vi "Determine Mouse Down Action.vi"(8 "error in (no error)":errorcluster, 11 "DataGrid in":refnum<class "DataGrid.lvclass">) -> (0 "error out":errorcluster, 2 "Action":T1, 3 "DataGrid out":refnum<class "DataGrid.lvclass">)   [LabVIEW 2017, in "DataGrid.lvclass"]
uses:
  DataGrid.lvclass
  C:/Program Files (x86)/National Instruments/LabVIEW 2017/vi.lib/QSI/QControls/QControl Classes/MulticolumnListbox/MulticolumnListbox.lvclass
  Mouse Down Action.ctl
  Read Current Edit Position.vi
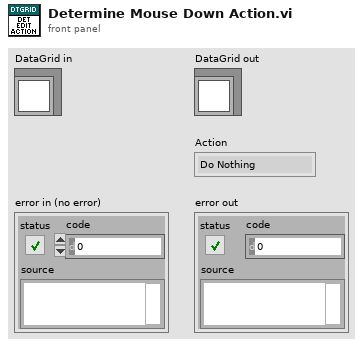
[diagram p1: front panel]
types:
  T1 = typedef "DataGrid.lvclass/Mouse Down Action.ctl" = enum16{"Do Nothing", "Sort Column", "Edit Only", "Add Row and Edit"}
  T2 = typedef "LVRowAndColumnTypeDef.ctl" = cluster{"Row":i32, "Column":i32}
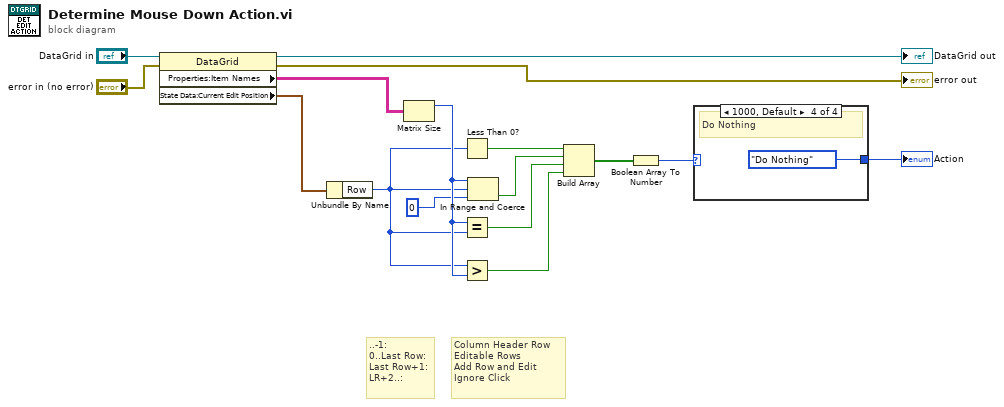
[diagram p0: block diagram]
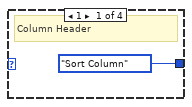
[diagram p2: hidden frame]
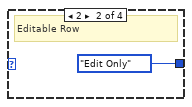
[diagram p3: hidden frame]
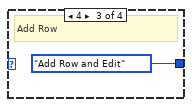
[diagram p4: hidden frame]
diagram:
  # "Column Header Row\nEditable Rows\nAdd Row and Edit\nIgnore Click"
  # "..-1:\n0..Last Row:\nLast Row+1:\nLR+2..:"
  n1 = property class="DataGrid"(reference="DataGrid in", error in="error in (no error)") -> (reference out=→"DataGrid out":refnum<class "DataGrid.lvclass">, error out=→"error out":errorcluster, "Properties:Item Names"=w13:string[][], "State Data:Current Edit Position"=w16:T2)
  n2 = Unbundle By Name(w16) -> ("Row"=w6:i32)
  n3 = Matrix Size(0:w13) -> (1:w7:i32)  [unwired: 1 out]
  n4 = Less Than 0?(x=w6) -> (x < 0?=w8:bool)
  n5 = Equal?(x=w7, y=w6) -> (x = y?=w10:bool)
  n6 = Greater?(x=w6, y=w7) -> (0:w11:bool)
  n7 = In Range and Coerce(upper limit=w7, x=w6, lower limit=0) -> (In Range?=w9:bool)  [unwired: 1 out]
  n8 = Build Array(w8, w9, w10, w11) -> (w12:bool[])
  n9 = Boolean Array To Number(Boolean array=w12) -> (number=w2:u32)
  n10 = case shown="1000, Default" w2 {
    tunnel: [Mouse_Down_Action."Sort Column" ("Action") Mouse_Down_Action."Edit Only" ("Action") Mouse_Down_Action."Add Row and Edit" ("Action") Mouse_Down_Action."Do Nothing" ("Action")] -> w1
    frame 1 {
      # "Column Header"
    }
    frame 2 {
      # "Editable Row"
    }
    frame 4 {
      # "Add Row"
    }
    frame 8, Default {
      # "Do Nothing"
    }
  }
  "Action" <- w1
